vi "Stoermeldepuffer loggen.vi"   [LabVIEW 2020, in "Stoerungen.lvlib"]
uses:
  Stoerungen.lvlib
  FGV Stoermeldungen Aktion.ctl
  Seiten/System Einstellungen V2/Aktioen FGV System.ctl
  FGV Stoerungsdatei Aktionen.ctl
  Allgemein/allgemeine Sub-VIs.lvlib
  Seiten/System Einstellungen V2/System Einstellungen V2.lvlib
panel:
  # "Störmeldepuffer in Datei loggen!"
types:
  T1 = typedef "System Einstellungen V2.lvlib/Aktioen FGV System.ctl" = enum16{"lesen", "laden", "speichern", "Optionen schreiben", "Zeitstempel", "Reset BMP", "Reset SQP", "Wartung", "Werkseinstellung"}
  T2 = typedef "Stoerungen.lvlib/FGV Stoermeldungen Aktion.ctl" = enum16{"Initialisieren", "kommend", "gehend", "lesen", "Queue leeren", "Queue freigeben", "in Datei loggen", "Änderung zurücksetzen"}
  T3 = typedef "System Einstellungen V2.lvlib/Optionen.ctl" = cluster{"Störmeldep.":bool, "Betriebszustände":bool, "AK in ppm":bool, "log Cal-Gas":bool, "log 0-Gas":bool, "Durchflusssensor 0-5V":bool, "PNS?":bool, "Mit N2 spülen":bool, "TRE08":bool, "Amium 10-Fach":bool, "Verticale Scrollbar aktiv":bool, "Loggingtakt":bool, "AK Rezeptwechsel gleich wie MKS":bool, "NG ECO":bool}
  T4 = typedef "Stoerungen.lvlib/Stoermeldung.ctl" = cluster{"Zeitstempel":timestamp, "Nummer":i32, "Kommend":bool}
  T5 = typedef "Stoerungen.lvlib/FGV Stoerungsdatei Aktionen.ctl" = enum16{"lesen", "laden", "Neue Werte"}
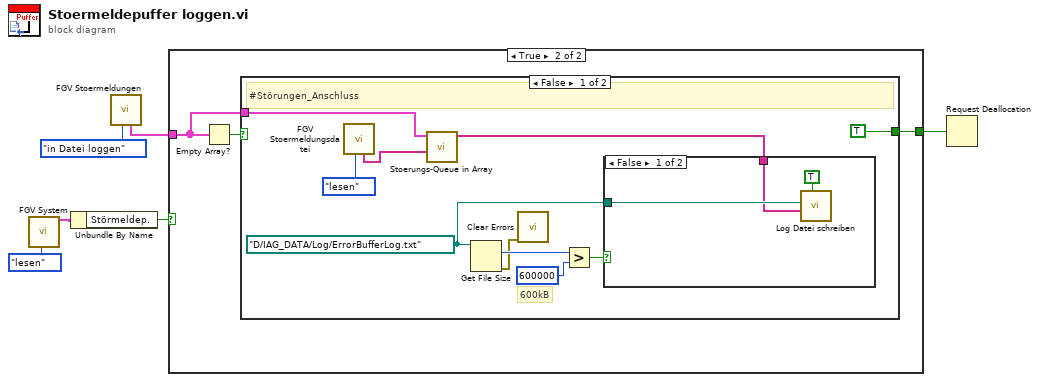
[diagram p0: block diagram]
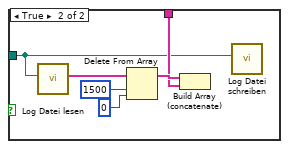
[diagram p3: hidden frame]
diagram:
  n1 = call "FGV System.vi"("Aktionen"=Aktioen_FGV_System."lesen") -> ("Optionen"=w3:T3)  [unwired: 12 in, 6 out]
  n2 = Unbundle By Name(w3) -> ("Störmeldep."=w2:bool)
  n3 = call "FGV Stoermeldungen.vi"("Aktion"=FGV_Stoermeldungen_Aktion."in Datei loggen") -> ("Loggen in Datei"=w5:T4[])  [unwired: 3 in, 7 out]
  n4 = case shown="True" w2 {
    tunnel: w5 -> [_ w8]
    tunnel: [_ w7] -> w1
    frame False {
    }
    frame True {
      n5 = Empty Array?(array=w8) -> (empty?=w9:bool)
      n6 = case shown="False" w9 {
        tunnel: w8 -> [w15 _]
        tunnel: [TRUE _] -> w7
        frame False {
          w13 = path "D:/IAG_DATA/Log/ErrorBufferLog.txt" ("Datei")
          # "600kB"
          # "#Störungen_Anschluss"
          n7 = call "FGV Stoermeldungsdatei.vi"("Aktionen"=FGV_Stoerungsdatei_Aktionen."lesen") -> ("Text"=w10:string[])  [unwired: 2 in, 8 out]
          n8 = call "Stoerungs-Queue in Array.vi"("Störmeldetexte aus Datei"=w10, "Queue-Inhalt (FGV Störmeldungen)"=w15) -> ("Tabelle Störmeldungen"=w14:string[])  [unwired: 9 in]
          n9 = Get File Size(file=w13) -> (size (in bytes)=w17:i64, 0:w12:errorcluster)  [unwired: 1 in, 1 out]
          n10 = call <vilib>:"Clear Errors.vi"("error in (no error)"=w12) -> ()  [unwired: 5 in, 2 out]
          n11 = Greater?(x=w17, y=i64 600000) -> (0:w19:bool)
          n12 = case shown="False" w19 {
            tunnel: w14 -> [w20 w25]
            tunnel: w13 -> [w21 w23]
            frame False {
              n13 = call "Log Datei schreiben.vi"("An Datei Anhängen?"=TRUE ("append to file? (new file:F)"), "Array"=w20, "Dateipfad"=w21) -> ()  [unwired: 8 in, 1 out]
            }
            frame True {
              n14 = call "Log Datei lesen.vi"("Dateipfad"=w23) -> ("Array"=w24:string[])  [unwired: 10 in]
              n15 = Delete From Array(array=w24, length=1500 ("Länge"), index=0 ("Index")) -> (array with subset deleted=w26:string[])  [unwired: 1 out]
              n16 = Build Array (concatenate)(w26, w25) -> ()  [unwired: 1 out]
              n17 = call "Log Datei schreiben.vi"("Dateipfad"=w23) -> ()  [unwired: 10 in, 1 out]
            }
          }
        }
        frame True {
        }
      }
    }
  }
  n18 = Request Deallocation(w1) -> ()
